vi "SCCT Start-Stop Service.vi"(8 "error out":errorcluster, 9 "Idle Time":u32=990, 10 "Publish Time":u32=5, 11 "publisher out":refnum<class "Publisher.lvclass">) -> (3 "publisher out 2":refnum<class "Publisher.lvclass">)   [LabVIEW 2011]
uses:
  <vilib>/TOOLS FOR SMART MINDS/SCCT/Publisher/Publisher.lvclass
  <vilib>/TOOLS FOR SMART MINDS/SCCT/Publisher/publishData_Message.vi
panel:
  in  "Stop Autonomous Mode":bool
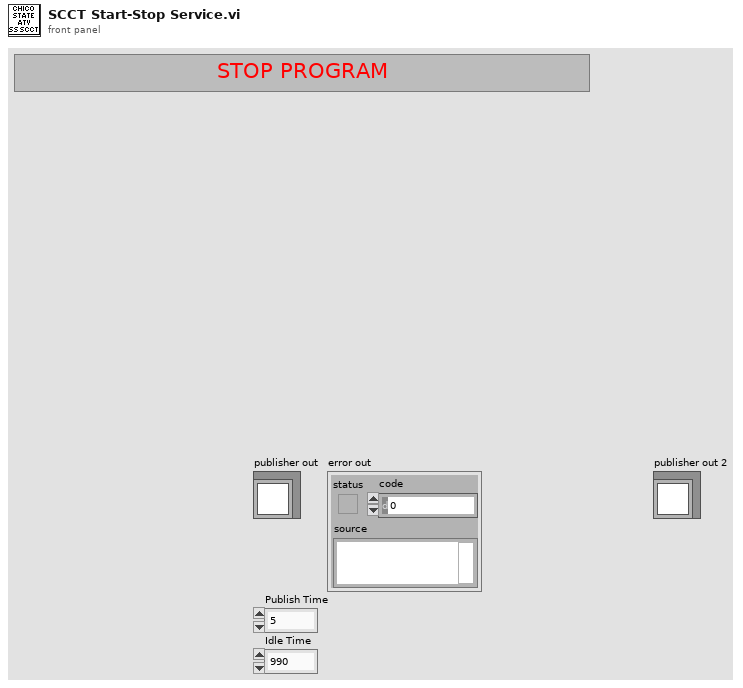
[diagram p1: front panel]
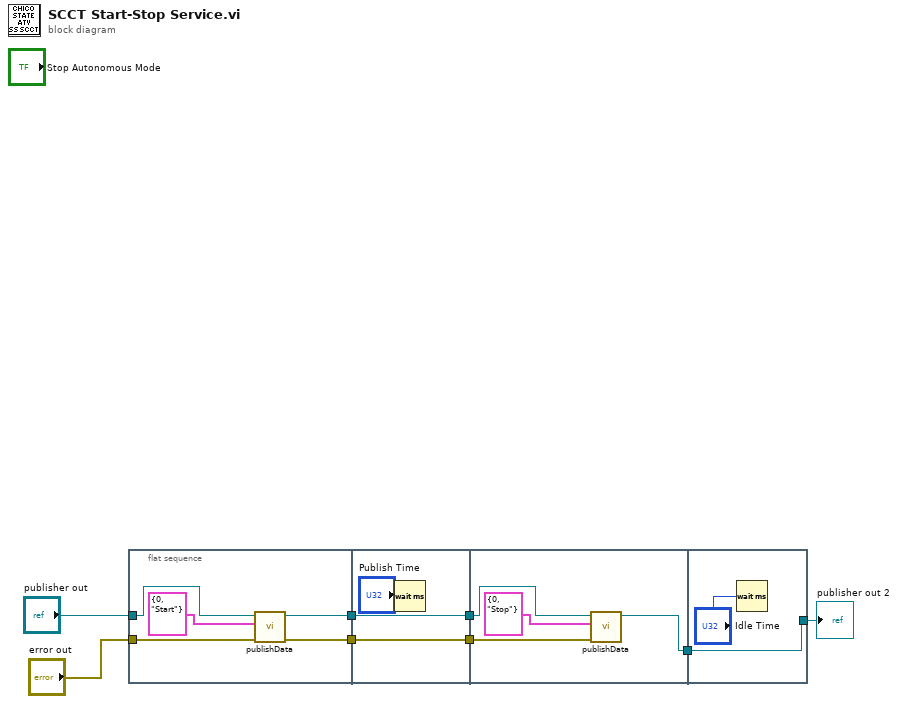
[diagram p0: block diagram]
diagram:
  n1 = flat-sequence {
    tunnel: "publisher out" -> [w12]
    tunnel: "error out" -> [w11]
    tunnel: [w10] -> w6
    tunnel: [w9] -> w5
    tunnel: w6 -> [w16]
    tunnel: w5 -> [w15]
    tunnel: [w16] -> w4
    tunnel: [w15] -> w3
    tunnel: w4 -> [w19]
    tunnel: w3 -> [w18]
    tunnel: [w17] -> w2
    tunnel: [w21] -> w1
    tunnel: w2 -> [w21]
    frame #0 {
      n2 = call-poly <vilib>:"publishData.vi"("error in (no error)"=w11, "value"=cluster{"code":i32, "description":string} {"code"=0, "description"="Start"}, "publisher in"=w12) -> ("error out"=w9:errorcluster, "publisher out"=w10:refnum<class "Publisher.lvclass">)  [unwired: 7 in]
    }
    frame #1 {
      n3 = Wait (ms)(milliseconds to wait="Publish Time") -> ()  [unwired: 1 out]
    }
    frame #2 {
      n4 = call-poly <vilib>:"publishData.vi"("error in (no error)"=w18, "value"=cluster{"code":i32, "description":string} {"code"=0, "description"="Stop"} ("value 2"), "publisher in"=w19) -> ("publisher out"=w17:refnum<class "Publisher.lvclass">)  [unwired: 7 in, 1 out]
    }
    frame #3 {
      n5 = Wait (ms)(milliseconds to wait="Idle Time") -> ()  [unwired: 1 out]
    }
  }
  "publisher out 2" <- w1
